vi "FSM.vi"() -> ()   [LabVIEW 2012]
panel:
  in  "stop":bool
  in  "Change Sequence":bool
  out "Stage 4":bool
  out "Stage 3":bool
  out "Stage 2":bool
  out "Stage 1":bool
  # "Finite State Machine"
  # "Stage 1"
  # "Stage 2"
  # "Change Sequence"
  # "Stage 3"
  # "Stage 4"
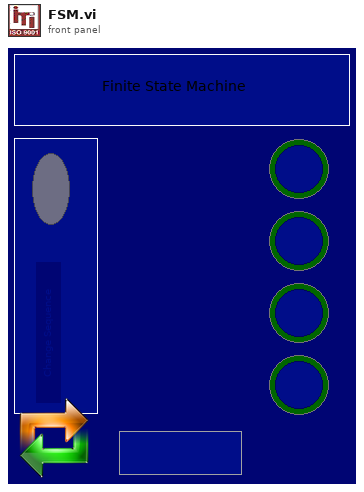
[diagram p1: front panel]
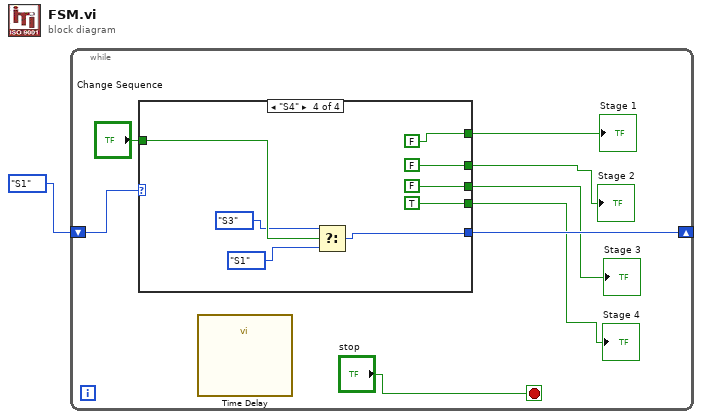
[diagram p0: block diagram]
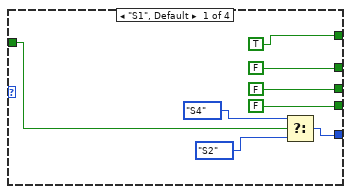
[diagram p2: hidden frame]
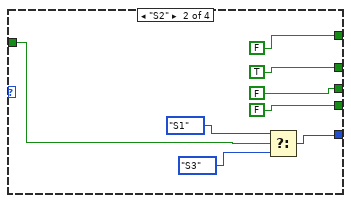
[diagram p3: hidden frame]
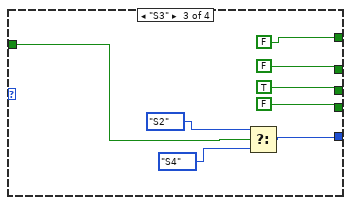
[diagram p4: hidden frame]
diagram:
  n1 = while {
    shift-right: [w7] -> _
    shift-left: enum16{"S1", "S2", "S3", "S4"}."S1" -> [w8]
    stop <- "stop" stop-if-true
    n2 = case shown="\"S4\"" w8 {
      tunnel: [w10 w19 w27 w34] -> w7
      tunnel: [TRUE FALSE FALSE FALSE] -> w6
      tunnel: [FALSE TRUE FALSE FALSE] -> w5
      tunnel: [FALSE FALSE TRUE FALSE] -> w4
      tunnel: [FALSE FALSE FALSE TRUE] -> w3
      tunnel: "Change Sequence" -> [w11 w18 w26 w37]
      frame "S1", Default {
        n3 = Select(t=enum16{"S1", "S2", "S3", "S4"}."S4", s=w11, f=enum16{"S1", "S2", "S3", "S4"}."S2") -> (s? t:f=w10:enum16{"S1", "S2", "S3", "S4"})
      }
      frame "S2" {
        n4 = Select(t=enum16{"S1", "S2", "S3", "S4"}."S1", s=w18, f=enum16{"S1", "S2", "S3", "S4"}."S3") -> (s? t:f=w19:enum16{"S1", "S2", "S3", "S4"})
      }
      frame "S3" {
        n5 = Select(t=enum16{"S1", "S2", "S3", "S4"}."S2", s=w26, f=enum16{"S1", "S2", "S3", "S4"}."S4") -> (s? t:f=w27:enum16{"S1", "S2", "S3", "S4"})
      }
      frame "S4" {
        n6 = Select(t=enum16{"S1", "S2", "S3", "S4"}."S3", s=w37, f=enum16{"S1", "S2", "S3", "S4"}."S1") -> (s? t:f=w34:enum16{"S1", "S2", "S3", "S4"})
      }
    }
    "Stage 1" <- w6
    "Stage 2" <- w5
    "Stage 3" <- w4
    "Stage 4" <- w3
    n7 = call "Time Delay"() -> ()  [unwired: 11 in, 1 out]
  }
